vi "Get Window DPI.vi"(8 "error in (no error)":errorcluster, 11 "window refnum (NaWR)":T1) -> (0 "error out":errorcluster, 2 "DPI":i32, 3 "window refnum out":T1)   [LabVIEW 2020, in "MacroAssert.lvlib" / "WINUTIL.lvlib"]
doc: "This VI will find the coordinates of the upper left and lower right corners of the window identified by the 'window refnum' parameter. Coordinate values are in pixels, relative to the upper left corner of the screen. The 'window refnum' can be obtained by using 'Get Window RefNum.vi'."
uses:
  WINUTIL.lvlib
  Window Refnum.ctl
  kernel32.dll
  user32.dll
  SHCore.dll
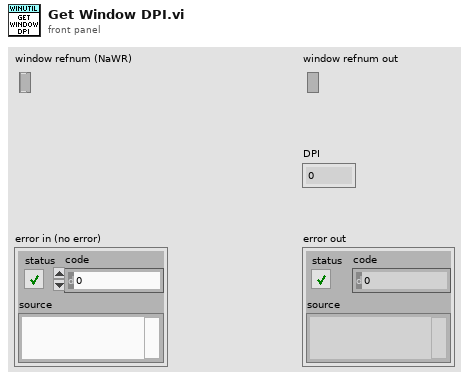
[diagram p1: front panel]
types:
  T1 = typedef "MacroAssert.lvlib/WINUTIL.lvlib/Window Refnum.ctl" = refnum<k1>
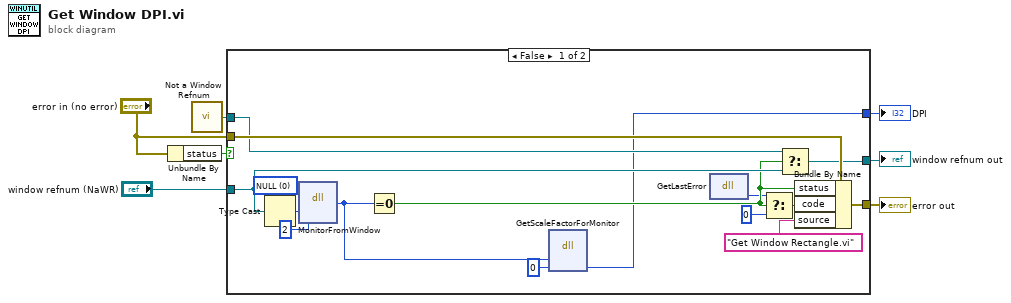
[diagram p0: block diagram]
diagram:
  n1 = Unbundle By Name("error in (no error)") -> ("status"=w7:bool)
  n2 = call "Not a Window Refnum.vi"() -> ("Not a Window Refnum"=w3:T1)
  n3 = case shown="False" w7 {
    tunnel: "error in (no error)" -> [w22 w25]
    tunnel: [w21 w24] -> w2
    tunnel: [w20 w25] -> w5
    tunnel: "window refnum (NaWR)" -> [w17 _]
    tunnel: w3 -> [w16 w24]
    tunnel: [w10 _] -> w1
    frame False {
      w18 = u32 0 items=["NULL"]
      n4 = Type Cast(type=w18, x=w17) -> (*(type *) &x=w19:u32)
      n5 = dll-call lib="USER32.DLL" fn="MonitorFromWindow" label="GetWindowRect"("hWnd"=w19, "dwFlags"=u32 2) -> ("Return Value"=w9:u32)  [unwired: 5 in, 2 out]
      n6 = Equal To 0?(x=w9) -> (x = 0?=w13:bool)
      n7 = dll-call lib="SHCore.dll" fn="GetScaleFactorForMonitor" label="GetWindowRect"("hMon"=w9, "pScale"=0) -> ("pScale"=w10:i32)  [unwired: 4 in, 3 out]
      n8 = dll-call lib="kernel32.dll" fn="GetLastError"() -> (w12:i32)  [unwired: 3 in, 2 out]
      n9 = Select(t=w12, s=w13, f=0) -> (s? t:f=w15:i32)
      n10 = Select(t=w16, s=w13, f=w17) -> (s? t:f=w21:T1)
      n11 = Bundle By Name(cluster=w22, "status"=w13, "code"=w15, "source"="Get Window Rectangle.vi") -> (w20:errorcluster)
    }
    frame True {
    }
  }
  "error out" <- w5
  "window refnum out" <- w2
  "DPI" <- w1
